vi "API.vi"   [LabVIEW 2021]
uses:
  LVCAM/LVCAM/Msg Strategy/Msg Strategy.lvclass
  LVCAM/Msgs/Actor Destroy/Actor Destroy Msg Strategy/Actor Destroy Msg Strategy.lvclass
  LVCAM/Msgs/Actor Last Ack/Actor Last Ack Msg Strategy/Actor Last Ack Msg Strategy.lvclass
  LVCAM/Msgs/Actor Create/Actor Create Msg Strategy/Actor Create Msg Strategy.lvclass
  LVCAM/LVCAM/Actor/Actor.lvclass
  LVCAM/LVCAM/Self Actor/Self Actor.lvclass
  LVCAM/Msgs/Actor Create/Actor Create/Actor Create.lvclass
  LVCAM/Msgs/Actor Last Ack/Actor Last Ack/Actor Last Ack.lvclass
  LVCAM/Msgs/Actor Destroy/Actor Destroy/Actor Destroy.lvclass
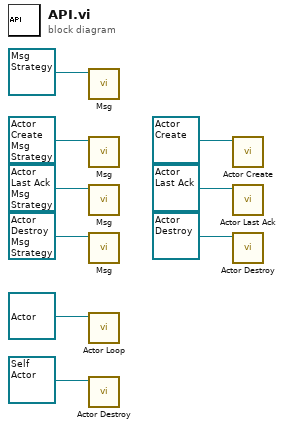
[diagram p0: block diagram]
diagram:
  n1 = call-dynamic "Msg.vi"("Msg Strategy in"=refnum<class "Msg Strategy.lvclass"> refnum ("Artifex Actor Model.lvlib:Msg.lvclass")) -> ()  [unwired: 9 in, 2 out]
  n2 = call-dynamic "Msg.vi"("Actor Create Msg Strategy in"=refnum<class "Actor Create Msg Strategy.lvclass"> refnum ("Artifex Actor Model.lvlib:Create Msg.lvclass")) -> ()  [unwired: 9 in, 2 out]
  n3 = call-dynamic "Msg.vi"("Actor Last Ack Msg Strategy in"=refnum<class "Actor Last Ack Msg Strategy.lvclass"> refnum ("Artifex Actor Model.lvlib:Last Ack Msg.lvclass")) -> ()  [unwired: 9 in, 2 out]
  n4 = call-dynamic "Msg.vi"("Actor Destroy Msg Strategy in"=refnum<class "Actor Destroy Msg Strategy.lvclass"> refnum ("Artifex Actor Model.lvlib:Destroy Msg.lvclass")) -> ()  [unwired: 9 in, 2 out]
  n5 = call "Actor Loop.vi"("Actor in"=refnum<class "Actor.lvclass"> refnum ("Artifex Actor Model.lvlib:Actor.lvclass")) -> ()  [unwired: 10 in, 1 out]
  n6 = call-dynamic "Actor Destroy.vi"("Self Actor in"=refnum<class "Self Actor.lvclass"> refnum ("Artifex Actor Model.lvlib:Self Actor.lvclass")) -> ()  [unwired: 9 in, 2 out]
  n7 = call-dynamic "Actor Create.vi"("Actor Create in"=refnum<class "Actor Create.lvclass"> refnum ("Create.lvlib:Create.lvclass")) -> ()  [unwired: 9 in, 2 out]
  n8 = call-dynamic "Actor Last Ack.vi"("Actor Last Ack in"=refnum<class "Actor Last Ack.lvclass"> refnum ("Last Ack.lvlib:Last Ack.lvclass")) -> ()  [unwired: 9 in, 2 out]
  n9 = call-dynamic "Actor Destroy.vi"("Actor Destroy in"=refnum<class "Actor Destroy.lvclass"> refnum ("Destroy.lvlib:Destroy.lvclass")) -> ()  [unwired: 9 in, 2 out]
